vi "to string.vi"(8 "error in":errorcluster, 11 "Scan Engine configuration in":refnum<class "Scan Engine configuration.lvclass">) -> (0 "error out":errorcluster, 1 "data":string, 2 "version":string, 3 "Scan Engine configuration out":refnum<class "Scan Engine configuration.lvclass">)   [LabVIEW 2013, in "Scan Engine configuration.lvclass"]
doc: "Provides an interface for saving a module configuration to a file or other serialized data source. It is recommended that all children of this class store data in two sets--data required for its own initialization, and any data required for parent initialization--and that each implementation uses the <b>Call Parent Method</b> primitive to serialize parent information."
uses:
  Scan Engine configuration.lvclass
  <vilib>/NI/Tag Bus Module Framework/module configuration/TBM module configuration.lvclass
  Scan Engine configuration.lvclass/Scan Engine configuration.ctl
  current version.vi
  <vilib>/NI/Tag Bus Module Framework/root configuration/TBM configuration.lvclass
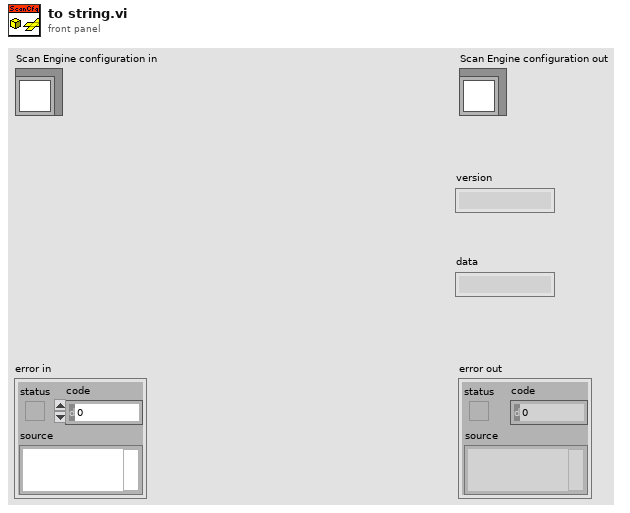
[diagram p1: front panel]
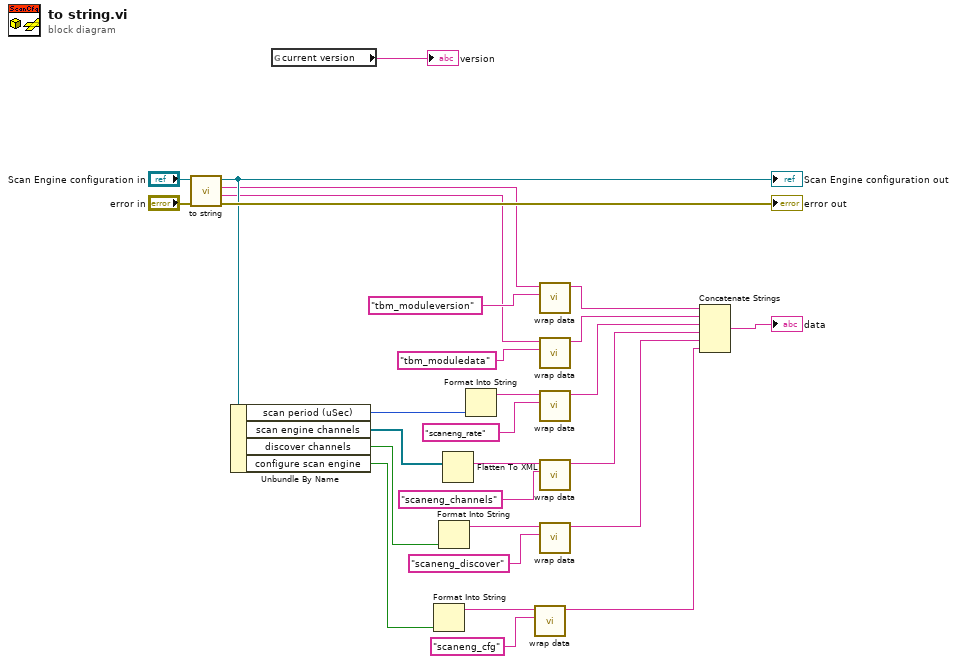
[diagram p0: block diagram]
diagram:
  n1 = call-parent "to string.vi"("error in"="error in", "module configuration in"="Scan Engine configuration in") -> ("error out"=→"error out":errorcluster, "data"=w15:string, "version"=w16:string, "module configuration out"=w17:refnum<class "Scan Engine configuration.lvclass">)  [unwired: 6 in]
  "Scan Engine configuration out" <- w17
  n2 = Unbundle By Name(w17) -> ("scan period (uSec)"=w13:u32, "scan engine channels"=w14:refnum<class "TBM channel.lvclass">[], "discover channels"=w8:bool, "configure scan engine"=w2:bool)
  n3 = global read "current version.vi" "current version"() -> (→"version":string)
  n4 = Format Into String(w2) -> (resulting string=w3:string)  [unwired: 3 in, 1 out]
  n5 = Format Into String(w8) -> (resulting string=w7:string)  [unwired: 3 in, 1 out]
  n6 = Flatten To XML(anything=w14) -> (xml string=w20:string)
  n7 = Format Into String(w13) -> (resulting string=w12:string)  [unwired: 3 in, 1 out]
  n8 = call <vilib>:"wrap data.vi"("identifier"="scaneng_cfg" ("additional identifier"), "data to wrap"=w3) -> ("wrapped data"=w1:string)  [unwired: 9 in]
  n9 = call <vilib>:"wrap data.vi"("identifier"="tbm_moduleversion" ("additional identifier"), "data to wrap"=w16) -> ("wrapped data"=w22:string)  [unwired: 9 in]
  n10 = call <vilib>:"wrap data.vi"("identifier"="tbm_moduledata" ("additional identifier"), "data to wrap"=w15) -> ("wrapped data"=w21:string)  [unwired: 9 in]
  n11 = call <vilib>:"wrap data.vi"("identifier"="scaneng_rate" ("additional identifier"), "data to wrap"=w12) -> ("wrapped data"=w10:string)  [unwired: 9 in]
  n12 = call <vilib>:"wrap data.vi"("identifier"="scaneng_channels" ("additional identifier"), "data to wrap"=w20) -> ("wrapped data"=w19:string)  [unwired: 9 in]
  n13 = call <vilib>:"wrap data.vi"("identifier"="scaneng_discover" ("additional identifier"), "data to wrap"=w7) -> ("wrapped data"=w5:string)  [unwired: 9 in]
  n14 = Concatenate Strings(w22, w21, w10, w19, w5, w1) -> (→"data":string)
